vi "Set Number Of Steps.vi"(10 "Number Of Steps":T1, 11 "Model in":refnum<class "Model.lvclass">) -> (3 "Model out":refnum<class "Model.lvclass">)   [LabVIEW 2016, in "Model.lvclass"]
uses:
  Model.lvclass
  Typedefs/Number Of Steps.ctl
  Model.lvclass/Model.ctl
  Typedefs/HPMT_Typedefs.lvlib
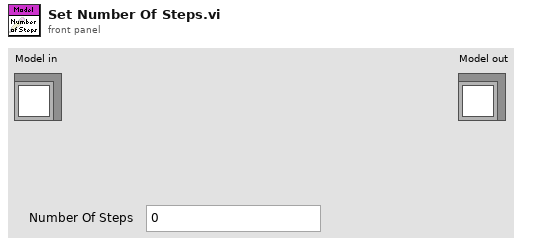
[diagram p1: front panel]
types:
  T1 = typedef "HPMT_Typedefs.lvlib/Number Of Steps.ctl" = i32
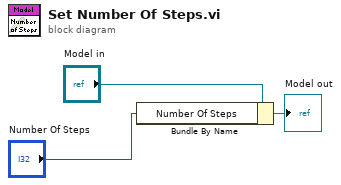
[diagram p0: block diagram]
diagram:
  n1 = Bundle By Name(cluster="Model in", "Number Of Steps"="Number Of Steps") -> (→"Model out":refnum<class "Model.lvclass">)
